vi "Init.vi"(8 "error in (no error)":errorcluster, 10 "Instrument String":variant, 11 "Lambda Gen LAN in":refnum<class "Lambda Gen LAN.lvclass">) -> (0 "error out":errorcluster, 2 "Found?":bool, 3 "Lambda Gen LAN out":refnum<class "Lambda Gen LAN.lvclass">)   [LabVIEW 2025, in "Power Supply.lvlib" / "Lambda Gen LAN.lvclass"]
uses:
  Lambda Gen LAN.lvclass
  Users/Public/Documents/Sandia National Labs/TSS Plugin/Abstract Engine.lvlibp/Plugin/Abstract/Instrument configuration/Instrument configuration.lvclass
  Lambda Gen LAN.lvclass/Lambda Gen LAN.ctl
  Users/Public/Documents/Sandia National Labs/TSS Plugin/Abstract Engine.lvlibp/Plugin/Abstract/Instrument configuration/Read Instrument Setting.vi
  Users/Public/Documents/Sandia National Labs/TSS Plugin/CEF.lvlibp/serializable configuration/CEF_serializable configuration.lvclass
  <instrlib>/TDK-Lambda GEN LAN Series/TDK-Lambda GEN LAN Series.lvlib
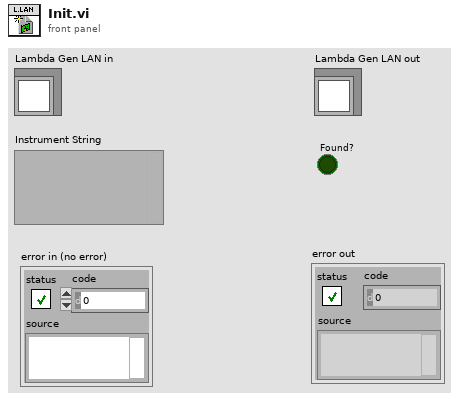
[diagram p1: front panel]
types:
  T1 = typedef "Abstract Engine.lvlibp/Instrument configuration.lvclass/Default Instrument.ctl" = cluster{"Type":string, "Address":string, "SW Alias":string, "Description":string, "Enabled":bool}
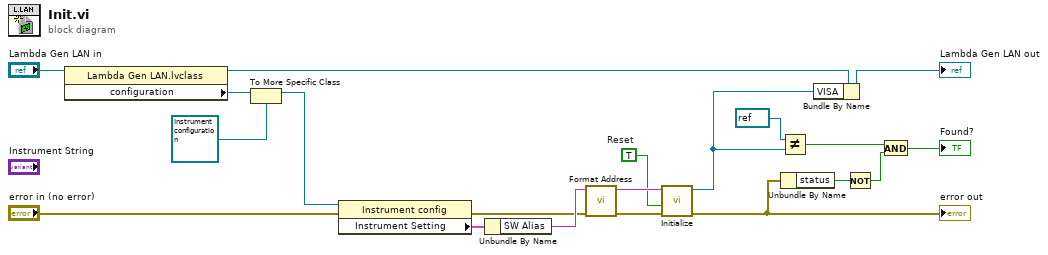
[diagram p0: block diagram]
diagram:
  w1 = TRUE  # Reset
  n1 = property class="Lambda Gen LAN.lvclass"(reference="Lambda Gen LAN in") -> (reference out=w12:refnum<class "Lambda Gen LAN.lvclass">, "configuration"=w14:refnum<class "CEF_serializable configuration.lvclass">)  [unwired: 1 in, 1 out]
  n2 = To More Specific Class(target class=refnum<class "Instrument configuration.lvclass"> refnum ("Abstract PlugIn.lvlibp:Instrument configuration"), reference=w14) -> (specific class reference=w15:refnum<class "Instrument configuration.lvclass">)  [unwired: 1 in, 1 out]
  n3 = property class="Instrument config"(reference=w15, error in="error in (no error)") -> (error out=w9:errorcluster, "Instrument Setting"=w2:T1)  [unwired: 1 out]
  n4 = Unbundle By Name(w2) -> ("SW Alias"=w11:string)
  n5 = call "Format Address.vi"("error in (no error)"=w9, "Address"=w11) -> ("error out"=w19:errorcluster, "Formatted Address"=w18:string)  [unwired: 8 in]
  n6 = call <instrlib>:"Initialize.vi"("error in (no error)"=w19, "Reset (T)"=w1, "VISA name"=w18) -> ("error out"=w7:errorcluster, "VISA out"=w16:refnum<visa-resource-name>)  [unwired: 7 in]
  "error out" <- w7
  n7 = Not Equal?(x=refnum<visa-resource-name> refnum ("VISA out"), y=w16) -> (x != y?=w6:bool)
  n8 = Unbundle By Name(w7) -> ("status"=w8:bool)
  n9 = Bundle By Name(cluster=w12, "VISA"=w16) -> (→"Lambda Gen LAN out":refnum<class "Lambda Gen LAN.lvclass">)
  n10 = Not(x=w8) -> (.not. x?=w5:bool)
  n11 = And(x=w6, y=w5) -> (x .and. y?=→"Found?":bool)
